vi "uTTA_SetCH_Description.vi"(4 "error in":errorcluster, 5 "Channel No":i32, 6 "Channel Description":T2, 7 "VISA Refnum in":refnum<visa-resource-name>) -> (0 "error out":errorcluster, 2 "Received":string, 3 "VISA Refnum out":refnum<visa-resource-name>)   [LabVIEW 2021]
uses:
  uTTA_Controls/CTL_uTTA_TSP_CalStatus.ctl
  uTTA_Controls/GV_uTTA_Configuration.vi
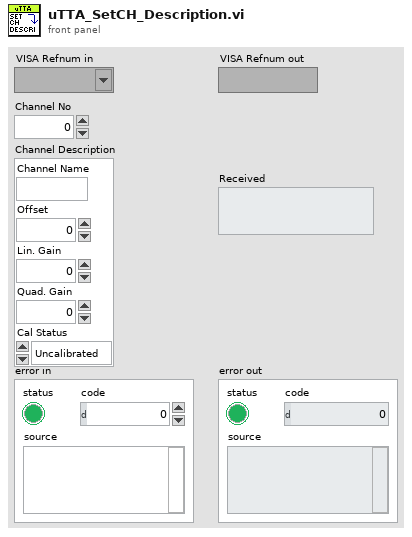
[diagram p1: front panel]
types:
  T1 = typedef "CTL_uTTA_TSP_CalStatus.ctl" = enum16{"Uncalibrated", "Calibrated", "Dummy"}
  T2 = cluster{"Channel Name":string, "Offset":dbl, "Lin. Gain":dbl, "Quad. Gain":dbl, "Cal Status":T1}
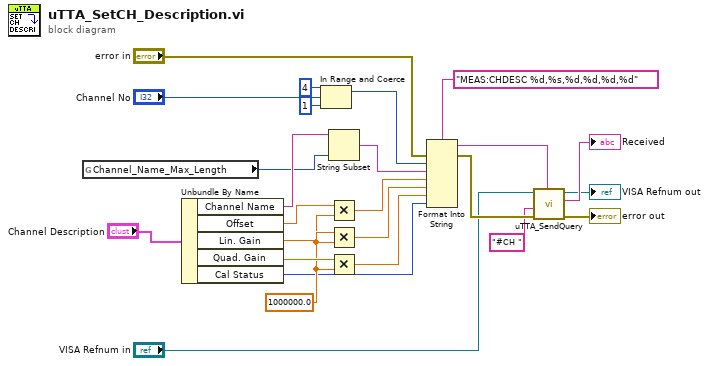
[diagram p0: block diagram]
diagram:
  w5 = 1000000.0 ("y")
  n1 = global read "GV_uTTA_Configuration.vi" "Channel_Name_Max_Length"() -> (w1:u32)
  n2 = Unbundle By Name("Channel Description") -> ("Channel Name"=w12:string, "Offset"=w11:dbl, "Lin. Gain"=w7:dbl, "Quad. Gain"=w6:dbl, "Cal Status"=w2:T1)
  n3 = In Range and Coerce(upper limit=4, x="Channel No", lower limit=1) -> (coerced(x)=w15:i32)  [unwired: 1 out]
  n4 = String Subset(string=w12, length (rest)=w1) -> (substring=w17:string)  [unwired: 1 in]
  n5 = Multiply(x=w11, y=w5) -> (x*y=w10:dbl)
  n6 = Multiply(x=w7, y=w5) -> (x*y=w9:dbl)
  n7 = Multiply(x=w6, y=w5) -> (x*y=w8:dbl)
  n8 = Format Into String(format string="MEAS:CHDESC %d,%s,%d,%d,%d,%d", error in="error in", w15, w17, w10, w9, w8, w2) -> (resulting string=w22:string, error out=w24:errorcluster)  [unwired: 1 in]
  n9 = call "uTTA_SendQuery.vi"("Send String"=w22, "error in (no error)"=w24, "Response Qualifier(\"\")"="#CH " ("Response Qualifier(\"\")"), "VISA Refnum in"="VISA Refnum in") -> ("error out"=→"error out":errorcluster, "Received"=→"Received":string, "VISA Refnum out"=→"VISA Refnum out":refnum<visa-resource-name>)  [unwired: 5 in]
